vi "Commascript advanced - Copy.vi"() -> ()   [LabVIEW 2017]
panel:
  in  "Starting Pos":i16(slide)=128 scale=340.0..50.0
  in  "string":string
  out "new picture":picture
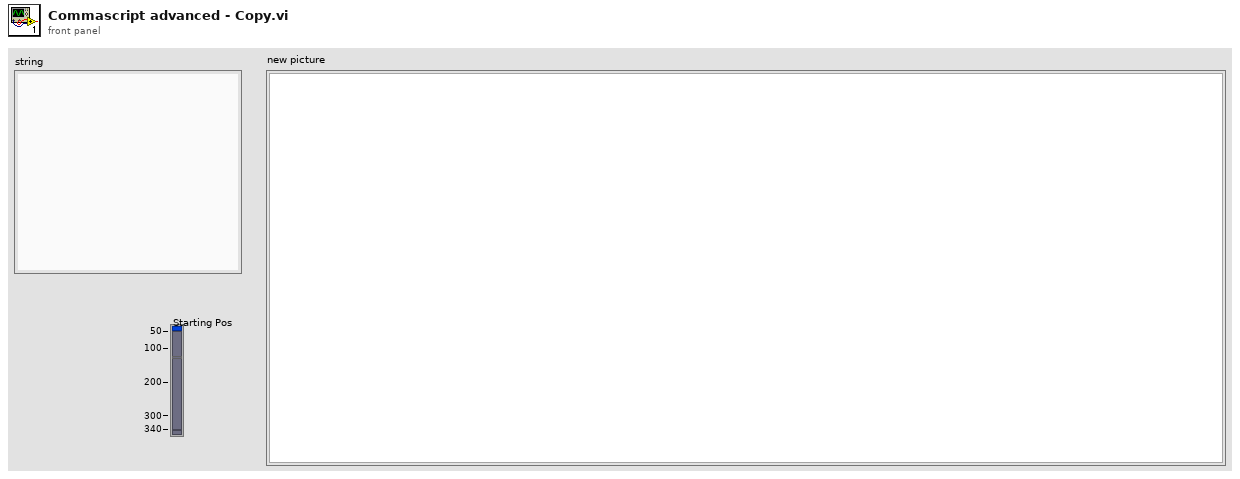
[diagram p1: front panel]
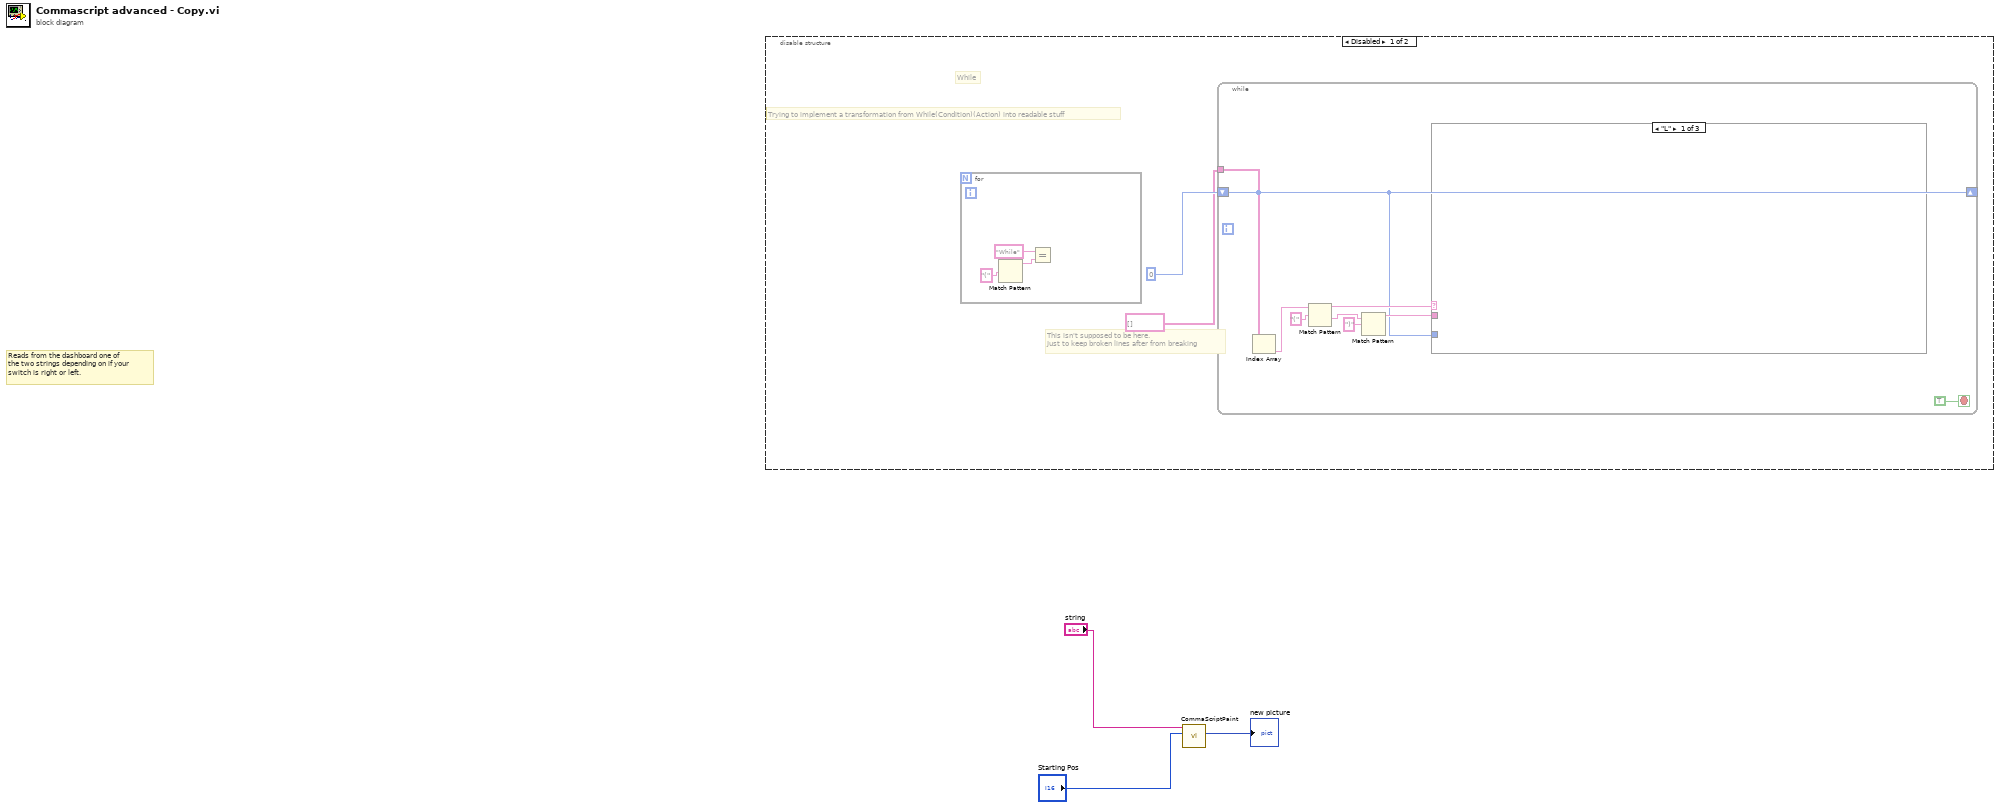
[diagram p0: block diagram]
diagram:
  # "Reads from the dashboard one of\nthe two strings depending on if your\nswitch is right or left."
  n1 = disable-structure shown="Disabled" {
    frame Disabled {
      # "While"
      # "This isn't supposed to be here.\nJust to keep broken lines after from breaking"
      # "Trying to implement a transformation from While(Condition)(Action) into readable stuff"
      n2 = for {
        n3 = Match Pattern(regular expression="(") -> (before substring=w7:string)  [unwired: 2 in, 3 out]
        n4 = Equal?(x="While", y=w7) -> ()  [unwired: 1 out]
      }
      n5 = while {
        tunnel: string[] [] -> [w13]
        shift-right: [w9] -> _
        shift-left: 0 -> [w9]
        stop <- TRUE stop-if-true
        n6 = Index Array(array=w13, index=w9) -> (element=w12:string)
        n7 = Match Pattern(string=w12, regular expression="(") -> (before substring=w11:string, after substring=w16:string)  [unwired: 1 in, 2 out]
        n8 = Match Pattern(string=w16, regular expression=")") -> (before substring=w10:string)  [unwired: 1 in, 3 out]
        n9 = case shown="\"L\"" w11 {
          tunnel: w10 -> [_ _ _]
          tunnel: w9 -> [_ _ _]
          frame "L" {
          }
          frame "D", Default {
          }
          frame "R" {
          }
        }
      }
    }
    frame Enabled {
    }
  }
  n10 = call "CommaScriptPaint.vi"("Starting Pos"="Starting Pos", "string"="string") -> ("new picture"=→"new picture":picture)  [unwired: 8 in, 1 out]
